vi "Init Panels.vi"(8 "error in (no error)":errorcluster, 11 "Entity Editor in":refnum<class "Entity Editor.lvclass">) -> (0 "error out":errorcluster, 3 "Entity Editor out":refnum<class "Entity Editor.lvclass">)   [LabVIEW 2020, in "Conditum-Tools.lvlib" / "Entity Editor.lvclass"]
uses:
  Entity Editor.lvclass
  <vilib>/IlluminatedG/IG OOPanel/OOPanel/ArrayManager/ArrayManager.lvclass
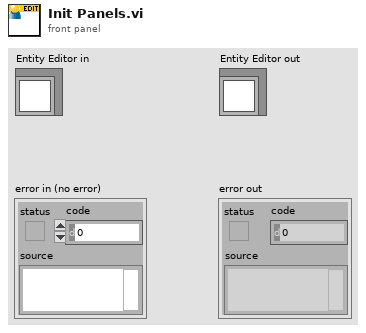
[diagram p1: front panel]
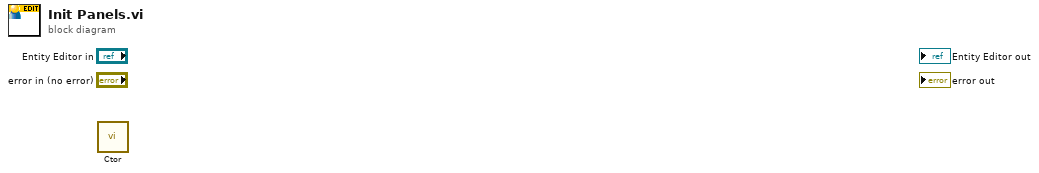
[diagram p0: block diagram]
diagram:
  n1 = call <vilib>:"Ctor.vi"() -> ()  [unwired: 10 in, 2 out]
